vi "超标留样启动运行.vi"(8 "error in (no error)":errorcluster) -> (0 "error out":errorcluster)   [LabVIEW 2016, in "德润DR803M超标留样.lvlib"]
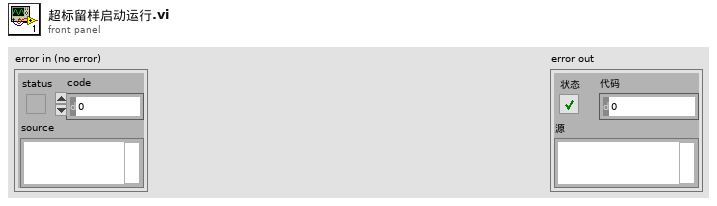
[diagram p1: front panel]
types:
  T1 = cluster{"STEP":enum16{"open", "read", "write", "close"}, "写入缓冲区":string}
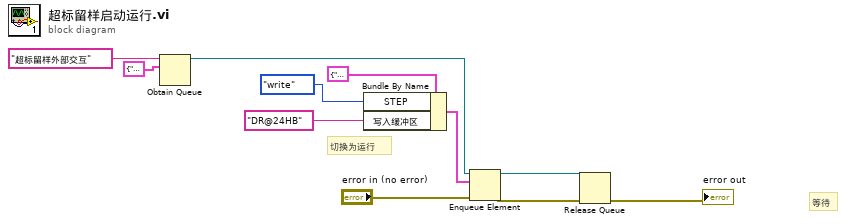
[diagram p0: block diagram]
diagram:
  # "等待"
  # "切换为运行"
  n1 = Obtain Queue(name (unnamed)="超标留样外部交互" ("名称（未命名）"), element data type=T1 {"STEP"=enum."write", "写入缓冲区"="ª\u0006\u0000\u0000P`\u00000»"}) -> (queue out=w9:refnum<queue>)  [unwired: 3 in, 2 out]
  n2 = Bundle By Name(cluster=T1 {"STEP"=enum."write", "写入缓冲区"="ª\u0006\u0000\u0000P`\u00000»"}, "STEP"=enum16{"open", "read", "write", "close"}."write", "写入缓冲区"="DR@24HB") -> (w4:T1)
  n3 = Enqueue Element(queue=w9, element=w4, error in (no error)="error in (no error)") -> (queue out=w2:refnum<queue>, error out=w3:errorcluster)  [unwired: 1 in, 1 out]
  n4 = Release Queue(queue=w2, error in (no error)=w3) -> (error out=→"error out":errorcluster)  [unwired: 1 in, 2 out]
